vi "Destroy.vi"(8 "error in (no error)":errorcluster, 11 "Ring buffer DVR":refnum<data-value>) -> (0 "error out":errorcluster)   [LabVIEW 2021, in "Ring Buffer Time Series Data.lvlib"]
uses:
  Ring Buffer Time Series Data.lvlib
  SubVIs/DVR data.ctl
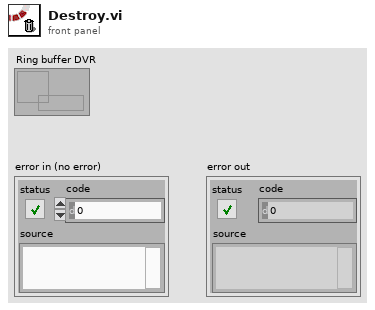
[diagram p1: front panel]
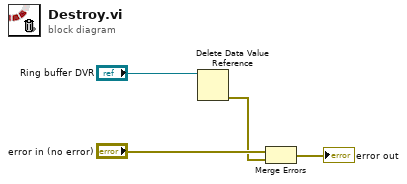
[diagram p0: block diagram]
diagram:
  n1 = Delete Data Value Reference(data value reference="Ring buffer DVR") -> (error out=w2:errorcluster)  [unwired: 1 in, 1 out]
  n2 = Merge Errors("error in (no error)", w2) -> (→"error out":errorcluster)
